vi "Get Waveform Bytes.vi"(11 "Waveforms":T1[](array[typedef])) -> (3 "Bytes":i32)   [LabVIEW 2021, in "ChannelCommon.lvlib"]
uses:
  ChannelCommon.lvlib
  typedef/Datatype Waveform.ctl
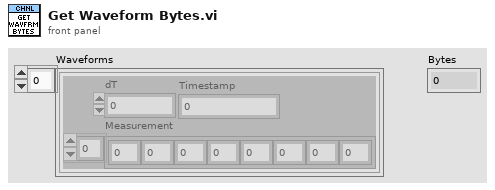
[diagram p1: front panel]
types:
  T1 = typedef "ChannelCommon.lvlib/Datatype Waveform.ctl" = cluster{"Measurement":dbl[], "dT":dbl, "Timestamp":i64}
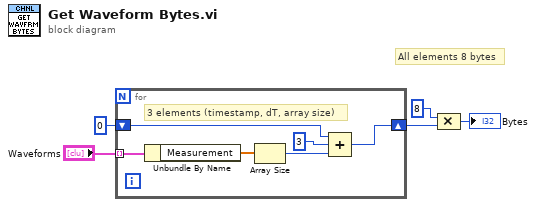
[diagram p0: block diagram]
diagram:
  # "All elements 8 bytes"
  n1 = for {
    tunnel: "Waveforms" -> [w11] mode=indexing
    shift-right: [w7] -> w3
    shift-left: 0 -> [w6]
    # "3 elements (timestamp, dT, array size)"
    n2 = Unbundle By Name(w11) -> ("Measurement"=w10:dbl[])
    n3 = Array Size(array=w10) -> (size(s)=w9:i32)
    n4 = Compound Arithmetic op=ADD(w6, 3 ("value"), w9) -> (w7:i32)
  }
  n5 = Compound Arithmetic op=MULTIPLY(8 ("value"), w3) -> (→"Bytes":i32)
